vi "ramp_simple.vi"() -> ()   [LabVIEW 2015]
uses:
  BERTTA.dll
panel:
  out "element 2":dbl
  in  "T_sp":dbl=40.0
  in  "Tr":dbl=20.0
  in  "time_set":dbl=2.0
  out "element":i32
  in  "reset":i32=1
  in  "pause":i32=1
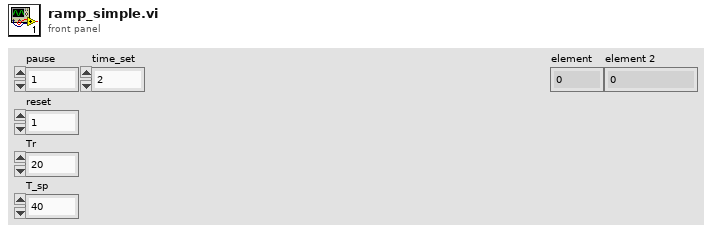
[diagram p1: front panel]
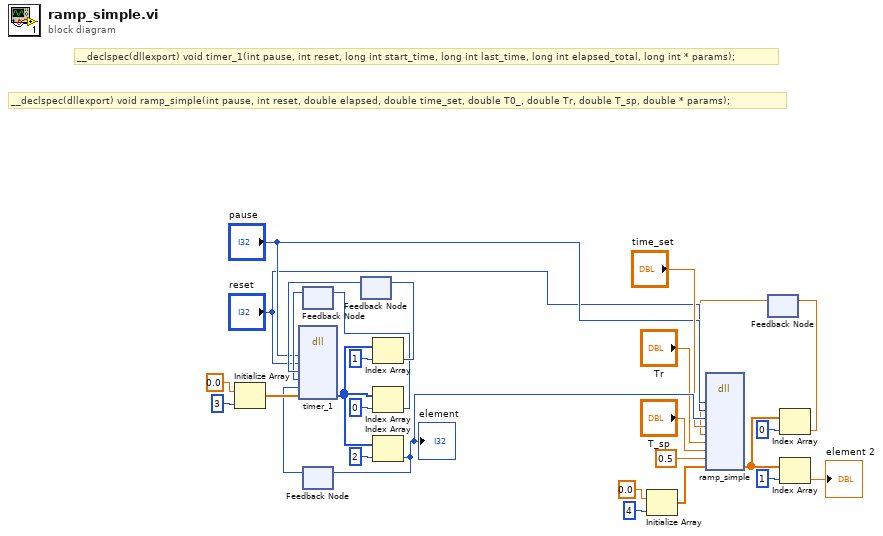
[diagram p0: block diagram]
diagram:
  # "__declspec(dllexport) void ramp_simple(int pause, int reset, double elapsed, double time_set, double T0_, double Tr, double T_sp, double * params);"
  # "__declspec(dllexport) void timer_1(int pause, int reset, long int start_time, long int last_time, long int elapsed_total, long int * params);"
  n1 = Initialize Array(0.0 ("element"), 3 ("dimension size")) -> (w28:dbl[])
  n2 = feedback #1() -> (w17:i32)  [unwired: 1 in]
  n3 = feedback #2() -> (w21:i32)  [unwired: 1 in]
  n4 = feedback #3() -> (w19:i32)  [unwired: 1 in]
  n5 = dll-call lib="C:/Users/shresplab/OneDrive - Kemira Oyj/Documents/Visual Studio 2017/Projects/Bertta/BERTTA/x64/Debug/BERTTA.dll" fn="timer_1"("pause"="pause", "reset"="reset", "start_time"=w19, "last_time"=w17, "elapsed_total"=w21, "params"=w28) -> ("params"=w22:i32[])  [unwired: 9 in, 2 out]
  n6 = Index Array(array=w22, index=1) -> (element=w20:i32)
  n7 = feedback-in #3(w20) -> ()
  n8 = Index Array(array=w22, index=0) -> (element=w18:i32)
  n9 = feedback-in #1(w18) -> ()
  n10 = Index Array(array=w22, index=2) -> (element=w16:i32)
  "element" <- w16
  n11 = feedback-in #2(w16) -> ()
  n12 = Initialize Array(0.0 ("element"), 4 ("dimension size")) -> (w13:dbl[])
  n13 = feedback #4() -> (w2:dbl)  [unwired: 1 in]
  n14 = dll-call lib="C:/Users/shresplab/OneDrive - Kemira Oyj/Documents/Visual Studio 2017/Projects/Bertta/BERTTA/x64/Debug/BERTTA.dll" fn="ramp_simple"("pause"="pause", "reset"="reset", "elapsed"=w16, "time_set"="time_set", "T0_"=w2, "Tr"="Tr", "T_sp"="T_sp", "treshold"=0.5, "params"=w13) -> ("params"=w4:dbl[])  [unwired: 12 in, 2 out]
  n15 = Index Array(array=w4, index=0) -> (element=w3:dbl)
  n16 = feedback-in #4(w3) -> ()
  n17 = Index Array(array=w4, index=1) -> (element=→"element 2":dbl)
